vi "Convert_DAC_to_Analog_channel.vi"(11 "Analog_IN":u16(slide) scale=1000.0..2000.0) -> (3 "DAC":u16)   [LabVIEW 2018]
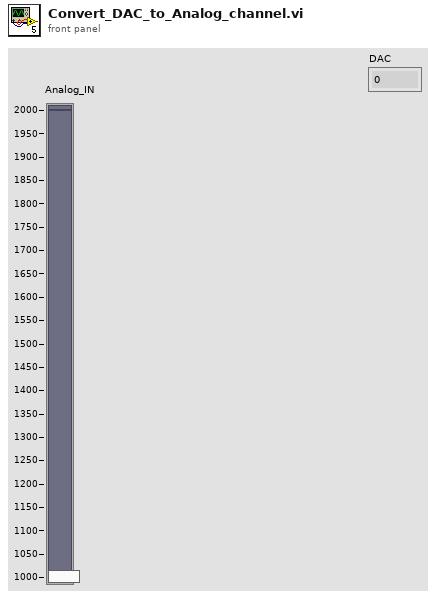
[diagram p1: front panel]
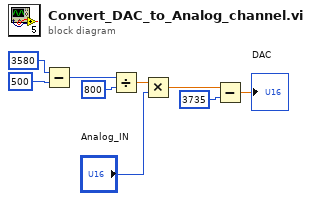
[diagram p0: block diagram]
diagram:
  n1 = Subtract(x=3580, y=500) -> (x-y=w6:i32)
  n2 = Divide(x=w6, y=800) -> (x/y=w1:dbl)
  n3 = Multiply(x=w1, y="Analog_IN") -> (x*y=w4:dbl)
  n4 = Subtract(x=w4, y=u16 3735) -> (x-y=→"DAC":dbl)
